vi "Obtain Request Events.vi"(8 "error in":errorcluster, 10 "Create New? (F)":bool, 11 "Module ID":i32=-1) -> (0 "error out":errorcluster, 2 "PLC Request Events":T1)   [LabVIEW 2024, in "PLC.lvlib"]
doc: "This VI Obtains/Creates the Requests events that will be used for other modules to communicate with the module that owns this VI. These Requests events will be accessed only via Public API methods for this module.\n\n<b>NOTE</b>: The contents of this VI are automatically generated and modified by the <b>Tools > DQMH Consortium > DQMH</b> utilities. Consider using those utilities instead of making your own modifications to this VI.\n_____\nBased on DQMH Dev Tools: Project Template 7.1.0.1503."
uses:
  PLC.lvlib
  Request Events--cluster.ctl
  Stop Argument--cluster.ctl
  Show Panel Argument--cluster.ctl
  Hide Panel Argument--cluster.ctl
  Show Diagram Argument--cluster.ctl
  Get Module Execution Status Argument--cluster.ctl
  Set IP Argument--cluster.ctl
  Connect Argument--cluster.ctl
  Connect (Reply Payload)--cluster.ctl
  Local Instance Request Events--cluster.ctl
  Wake Up HL Argument--cluster.ctl
  <vilib>/NI/Modbus Library/API/Master/Modbus Master.lvclass
  Local Instance Events SEQ/Local Instance Events SEQ.lvlib
panel:
  # "NOTE: The contents of this VI are automatically generated and modified by the Tools > DQMH Consortium > DQMH utilities. Consider using those utilities instead of making your own modifications to this VI."
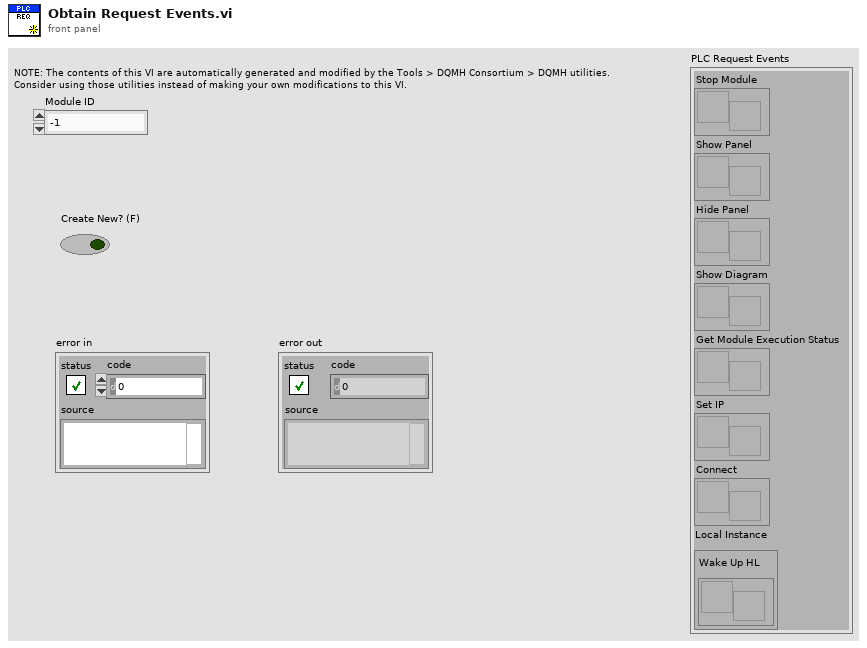
[diagram p1: front panel]
types:
  T1 = typedef "PLC.lvlib/Request Events--cluster.ctl" = cluster{"Stop Module":refnum<user-event>, "Show Panel":refnum<user-event>, "Hide Panel":refnum<user-event>, "Show Diagram":refnum<user-event>, "Get Module Execution Status":refnum<user-event>, "Set IP":refnum<user-event>, "Connect":refnum<user-event>, "Local Instance":T2}
  T2 = typedef "PLC.lvlib/Local Instance Request Events--cluster.ctl" = cluster{"Wake Up HL":refnum<user-event>}
  T3 = typedef "PLC.lvlib/Connect Argument--cluster.ctl" = cluster{"Module ID":i32, "Wait Notifier":refnum<notifier>, "wait for reply":bool}
  T4 = typedef "PLC.lvlib/Set IP Argument--cluster.ctl" = cluster{"Module ID":i32, "IP":string, "Port":i32}
  T5 = typedef "PLC.lvlib/Get Module Execution Status Argument--cluster.ctl" = cluster{"Module ID":i32, "Running?":bool}
  T6 = typedef "PLC.lvlib/Show Diagram Argument--cluster.ctl" = cluster{"Module ID":i32, "Debug?":bool}
  T7 = typedef "PLC.lvlib/Show Panel Argument--cluster.ctl" = cluster{"Module ID":i32, "Show Panel?":bool}
  T8 = typedef "PLC.lvlib/Hide Panel Argument--cluster.ctl" = cluster{"Module ID":i32, "Hide Panel?":bool}
  T9 = typedef "PLC.lvlib/Stop Argument--cluster.ctl" = cluster{"Module ID":i32, "Origin":string, "Exit via Stop Module Req?":bool, "Wait for Module to stop?":bool}
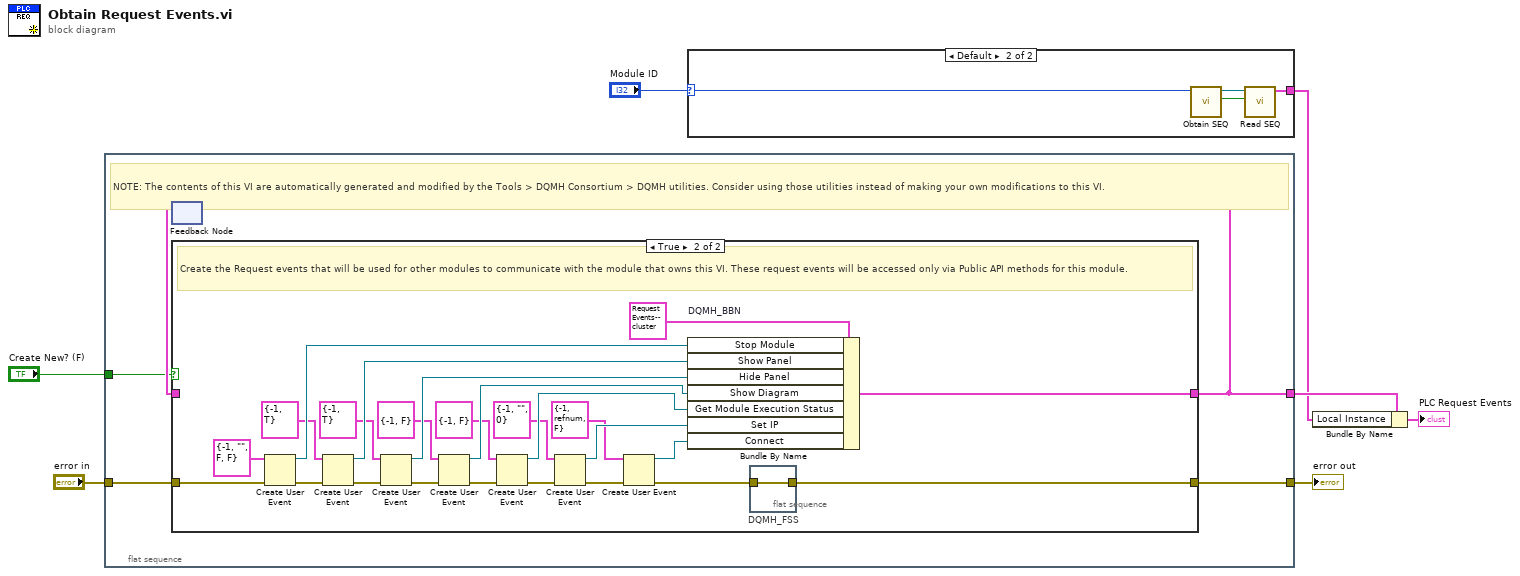
[diagram p0: block diagram]
diagram:
  n1 = flat-sequence {
    tunnel: [w12] -> w7
    tunnel: "error in" -> [w11]
    tunnel: [w9] -> w3
    tunnel: "Create New? (F)" -> [w8]
    frame #0 {
      # "NOTE: The contents of this VI are automatically generated and modified by the Tools > DQMH Consortium > DQMH utilities. Consider using those utilities instead of making your own modifications to this VI."
      n2 = feedback #1() -> (w10:T1)  [unwired: 1 in]
      n3 = case shown="True" w8 {
        tunnel: [w13 w27] -> w12
        tunnel: w11 -> [w13 w39]
        tunnel: [w14 w36] -> w9
        tunnel: w10 -> [w14 _]
        frame False {
        }
        frame True {
          # "Create the Request events that will be used for other modules to communicate with the module that owns this VI. These request events will be accessed only via Public API methods for this module."
          n4 = Create User Event(user event datatype=T9 {"Module ID"=-1, "Origin"="", "Exit via Stop Module Req?"=FALSE, "Wait for Module to stop?"=FALSE} ("Stop Argument"), error in=w39) -> (user event=w37:refnum<user-event>, error out=w34:errorcluster)
          n5 = Create User Event(user event datatype=T7 {"Module ID"=-1, "Show Panel?"=TRUE} ("Show Panel Argument"), error in=w34) -> (user event=w33:refnum<user-event>, error out=w31:errorcluster)
          n6 = Create User Event(user event datatype=T8 {"Module ID"=-1, "Hide Panel?"=TRUE} ("Hide Panel"), error in=w31) -> (user event=w30:refnum<user-event>, error out=w29:errorcluster)
          n7 = Create User Event(user event datatype=T6 {"Module ID"=-1, "Debug?"=FALSE} ("Show Diagram Argument"), error in=w29) -> (user event=w25:refnum<user-event>, error out=w26:errorcluster)
          n8 = Create User Event(user event datatype=T5 {"Module ID"=-1, "Running?"=FALSE} ("Get Module Execution Status Argument"), error in=w26) -> (user event=w22:refnum<user-event>, error out=w23:errorcluster)
          n9 = Create User Event(user event datatype=T4 {"Module ID"=-1, "IP"="", "Port"=0} ("Set IP Argument"), error in=w23) -> (user event=w19:refnum<user-event>, error out=w20:errorcluster)
          n10 = Create User Event(user event datatype=T3 {"Module ID"=-1, "Wait Notifier"=refnum, "wait for reply"=FALSE} ("Connect Argument"), error in=w20) -> (user event=w16:refnum<user-event>, error out=w17:errorcluster)
          n11 = Bundle By Name "DQMH_BBN"(cluster=T1 {"Stop Module"=refnum, "Show Panel"=refnum, "Hide Panel"=refnum, "Show Diagram"=refnum, "Get Module Execution Status"=refnum, "Set IP"=refnum, "Connect"=refnum, "Local Instance"={"Wake Up HL"=refnum}} ("output cluster"), "Stop Module"=w37, "Show Panel"=w33, "Hide Panel"=w30, "Show Diagram"=w25, "Get Module Execution Status"=w22, "Set IP"=w19, "Connect"=w16) -> (w36:T1)
          n12 = flat-sequence "DQMH_FSS" {
            tunnel: w17 -> [w40]
            tunnel: [w40] -> w27
            frame #0 {
            }
          }
        }
      }
      n13 = feedback-in #1(w9) -> ()
    }
  }
  n14 = case shown="Default" "Module ID" {
    selector: "Module ID" -> [_ w42]
    tunnel: [_ w41] -> w2
    frame -1 {
    }
    frame Default {
      n15 = call "Obtain SEQ.vi"("Module ID"=w42) -> ("Created New?"=w43:bool, "Local Instance Event SEQ"=w44:refnum<queue>)  [unwired: 8 in, 1 out]
      n16 = call "Read SEQ.vi"("Created New?"=w43, "Local Instance Event SEQ"=w44) -> ("Local Instance Request Events"=w41:T2)  [unwired: 8 in, 1 out]
    }
  }
  n17 = Bundle By Name(cluster=w3, "Local Instance"=w2) -> (→"PLC Request Events":T1)
  "error out" <- w7
